vi "Test Process Asynchronous Action Stopped when Process Stopped.vi"(8 "error in (no error)":errorcluster, 11 "Helper Loop Test In":refnum<class "Process Dev Test.lvclass">) -> (0 "error out":errorcluster, 3 "Helper Loop Test Out":refnum<class "Process Dev Test.lvclass">)   [LabVIEW 2020, in "Process Dev Test.lvclass"]
uses:
  source/Framework Test Suite/Mock Process/Mock Process.lvclass
  C:/Git/astemes-triarc-framework/source/Framework/Process/Process.lvclass
  source/Framework/Process/Process.lvclass/Process.ctl
  <vilib>/Astemes/LUnit/Test Case.lvclass/Test Case.ctl
  ff6210df-d80d-4043-ac84-bb28d4723d35.vi
  27698d7c-1d27-4f20-94d5-aa7beea38d40.vi
  3c03c699-6819-427c-a8c0-7eedb7611303.vi
  source/Framework/Process/Public/Lifecycle/Get Lifecycle State.vi
  source/Framework/Broadcast Event Helpers/Dequeue Broadcast Message by Message Cluster.vi
  <vilib>/Astemes/LUnit/Palette/Pass.vi
  <vilib>/Astemes/LUnit/Palette/Fail.vi
  <vilib>/Astemes/LUnit/Compare Variants.vi
  <vilib>/Astemes/LUnit/Describe Comparison.vi
  <vilib>/Astemes/LUnit/Set Assertion Type.vi
  source/Framework/Process/Private/SubVIs/Wait for finish.vi
  source/Framework/Process/Private/SubVIs/Set Lifecycle State.vi
  source/Framework/Process/Protected/Messaging/Send Message.vi
  <vilib>/Utility/error.llb/Clear Errors.vi
  source/Framework/Broadcast Event Helpers/Execution timer.vi
  <vilib>/Astemes/LUnit/Add test result.vi
  <vilib>/Astemes/LUnit/Variant to string.vi
  source/Framework/Process/Private/SubVIs/Handle Debug Data.vi
  <vilib>/Astemes/LUnit/LUnit Record Assertion Result.vi
  <vilib>/Utility/High Resolution Relative Seconds.vi
  <vilib>/Astemes/LUnit/LUnit Aggregate Assertion Results.vi
  <vilib>/Astemes/LUnit/Method Result/LUnit Merge Status.vi
  <vilib>/Astemes/LUnit/LUnit Concatenate result strings.vi
  <vilib>/Utility/error.llb/Error Cluster From Error Code.vi
  source/Framework/Broadcast Event Helpers/Dequeue Broadcast Message.vi
  <vilib>/Utility/Data Type/Get Type Information.vi
  <vilib>/Utility/LVClass/Get LV Class Name.vi
  source/Framework/Process/Process.lvclass
  Async Handling Test/Async Handling Test.lvclass/Async Handling Test.ctl
  Process Dev Test.lvclass
  Process Dev Test.lvclass/Process Dev Test.ctl
  C:/Git/astemes-triarc-framework/source/Framework/Base/Base.lvclass
  C:/Git/astemes-triarc-framework/source/Framework/Configuration File/Configuration File.lvclass
  C:/Git/astemes-triarc-framework/source/Framework/Configuration/Configuration.lvclass
  C:/Git/astemes-triarc-framework/source/Framework/Error Handler Interface/Error Handler Interface.lvclass
  C:/Git/astemes-triarc-framework/source/Framework/Logging/Logging.lvclass
  C:/Git/astemes-triarc-framework/source/Framework Test Suite/Mock Process/Mock Process.lvclass
  C:/Git/astemes-triarc-framework/source/Framework/Async Handler/Async Handler.lvclass
  C:/Git/astemes-triarc-framework/source/Framework/Helper Loop/Helper Loop.lvclass
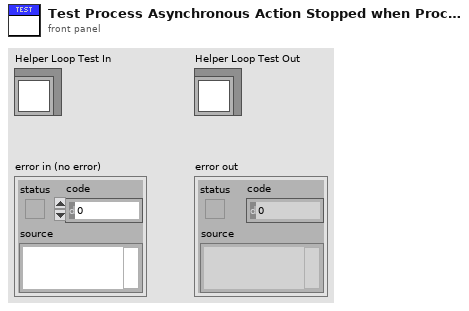
[diagram p1: front panel]
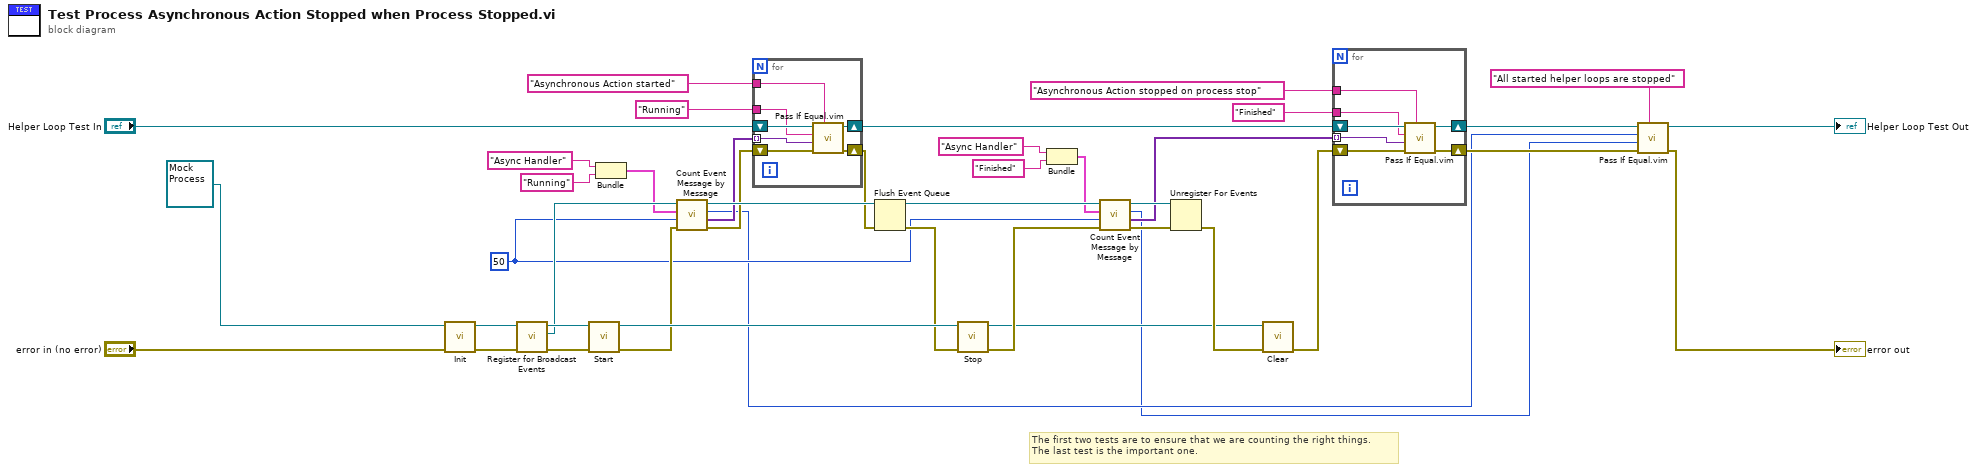
[diagram p0: block diagram]
diagram:
  w20 = 50 ("Timeout (-1)")
  # "The first two tests are to ensure that we are counting the right things. \nThe last test is the important one."
  n1 = call-dynamic "Init.vi"("error in (no error)"="error in (no error)", "Mock Process In"=refnum<class "Mock Process.lvclass"> refnum ("Mock Process.lvclass")) -> ("error out"=w36:errorcluster, "Mock Process Out"=w37:refnum<class "Mock Process.lvclass">)  [unwired: 8 in]
  n2 = call "Register for Broadcast Events.vi"("error in (no error)"=w36, "Process In"=w37) -> ("error out"=w34:errorcluster, "Event Registration Refnum Out"=w24:refnum<event-registration>, "Process Out"=w35:refnum<class "Mock Process.lvclass">)  [unwired: 7 in]
  n3 = call "Start.vi"("error in (no error)"=w34, "Process In"=w35) -> ("error out"=w22:errorcluster, "Process Out"=w33:refnum<class "Mock Process.lvclass">)  [unwired: 7 in, 1 out]
  n4 = Bundle("y"="Async Handler", "Description"="Running") -> (w4:cluster{"y":string, "Description":string})  [unwired: 1 in]
  n5 = call "Count Event Message by Message.vi"("error in (no error)"=w22, "Timeout"=w20, "Message"=w4, "Event Registration Refnum in"=w24) -> ("error out"=w19:errorcluster, "Message Data"=w15:variant[], "Count"=w10:i32, "Event Registration Refnum out"=w23:refnum<event-registration>)  [unwired: 4 in]
  n6 = for {
    tunnel: "Asynchronous Action started" ("Description") -> [w45]
    tunnel: "Running" ("Description") -> [w44]
    shift-right: [w49] -> w21
    shift-left: "Helper Loop Test In" -> [w48]
    shift-right: [w46] -> w18
    shift-left: w19 -> [w47]
    tunnel: w15 -> [w43] mode=indexing
    n7 = call "Pass If Equal.vim"("Description"=w45, "error in (no error)"=w47, "Actual"=w43, "Expected"=w44, "LUnit Test Case In"=w48) -> ("error out"=w46:errorcluster, "LUnit Test Case Out"=w49:refnum<class "Process Dev Test.lvclass">)  [unwired: 5 in]
  }
  n8 = Flush Event Queue(0:w23, 3:w18) -> (8:w29:refnum<event-registration>, 11:w28:errorcluster)  [unwired: 4 in, 1 out]
  n9 = call "Stop.vi"("error in (no error)"=w28, "Process In"=w33) -> ("error out"=w27:errorcluster, "Process Out"=w26:refnum<class "Mock Process.lvclass">)  [unwired: 7 in, 1 out]
  n10 = Bundle("y"="Async Handler", "Description"="Finished") -> (w1:cluster{"y":string, "Description":string})  [unwired: 1 in]
  n11 = call "Count Event Message by Message.vi"("error in (no error)"=w27, "Timeout"=w20, "Message"=w1, "Event Registration Refnum in"=w29) -> ("error out"=w25:errorcluster, "Message Data"=w14:variant[], "Count"=w9:i32, "Event Registration Refnum out"=w31:refnum<event-registration>)  [unwired: 4 in]
  n12 = Unregister For Events(event registration refnum=w31, error in=w25) -> (error out=w30:errorcluster)
  n13 = call-dynamic "Clear.vi"("error in (no error)"=w30, "Mock Process In"=w26) -> ("error out"=w32:errorcluster)  [unwired: 9 in]
  n14 = for {
    tunnel: w14 -> [w53] mode=indexing
    shift-right: [w54] -> w11
    shift-left: w32 -> [w56]
    shift-right: [w55] -> w12
    shift-left: w21 -> [w52]
    tunnel: "Asynchronous Action stopped on process stop" ("Description") -> [w51]
    tunnel: "Finished" ("Description") -> [w50]
    n15 = call "Pass If Equal.vim"("Description"=w51, "error in (no error)"=w56, "Actual"=w53, "Expected"=w50, "LUnit Test Case In"=w52) -> ("error out"=w54:errorcluster, "LUnit Test Case Out"=w55:refnum<class "Process Dev Test.lvclass">)  [unwired: 5 in]
  }
  n16 = call "Pass If Equal.vim"("Description"="All started helper loops are stopped", "error in (no error)"=w11, "Actual"=w9, "Expected"=w10, "LUnit Test Case In"=w12) -> ("error out"=→"error out":errorcluster, "LUnit Test Case Out"=→"Helper Loop Test Out":refnum<class "Process Dev Test.lvclass">)  [unwired: 5 in]
